vi "Get Motor Setpoint Value.vi"(8 "error in (no error)":errorcluster, 10 "state mode":T1 items=["undefined", "angle", "velocity"], 11 "motor communication in":refnum<class "NI_Robotics_Motor Communication Ref.lvclass">) -> (0 "error out":errorcluster, 1 "failed?":bool, 2 "value":dbl, 3 "motor communication out":refnum<class "NI_Robotics_Motor Communication Ref.lvclass">)   [LabVIEW 2017, in "NI_Robotics_Motor Communication Ref.lvclass"]
uses:
  <vilib>/robotics/Actuation/Motor Communication Ref/NI_Robotics_Motor Communication Ref.lvclass
  <vilib>/robotics/Actuation/Motor Communication/Motor State Mode.ctl
  <vilib>/robotics/Actuation/Motor Communication Ref/NI_Robotics_Motor Communication Ref.lvclass/NI_Robotics_Motor Communication Ref.ctl
  <vilib>/robotics/Actuation/Motor Communication/Read from Motor State.vi
  <vilib>/robotics/Actuation/Motor Communication/NI_Robotics_Motor Communication.lvclass
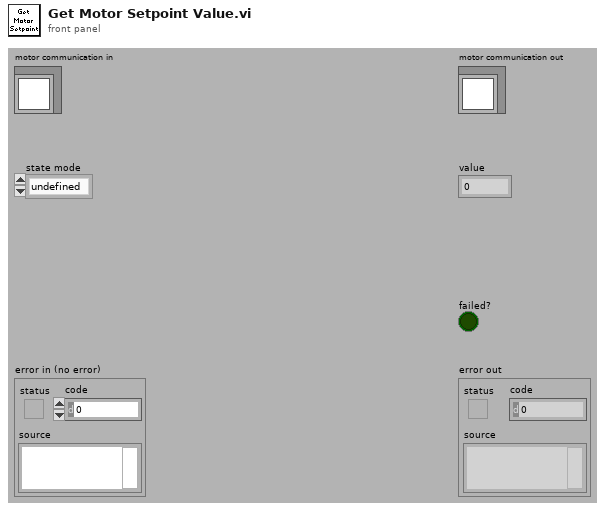
[diagram p1: front panel]
types:
  T1 = typedef "NI_Robotics_Motor Communication.lvclass/Motor State Mode.ctl" = u16
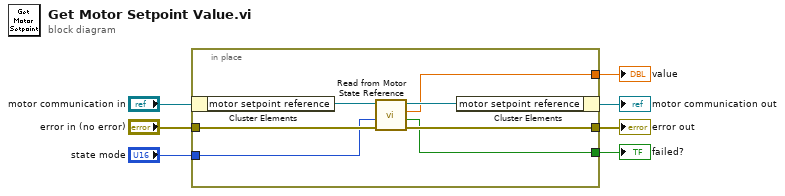
[diagram p0: block diagram]
diagram:
  n1 = in-place {
    in-place-border: [w12] -> w5
    in-place-border: "error in (no error)" -> [w11]
    in-place-border: [w10] -> w3
    in-place-border: [w9] -> w2
    in-place-border: "state mode" -> [w8]
    n2 = in-place-cluster #1("motor communication in") -> ("motor setpoint reference"=w14:refnum<data-value>)
    n3 = call <vilib>:"Read from Motor State Reference.vi"("error in (no error)"=w11, "state mode"=w8, "motor state ref in"=w14) -> ("error out"=w10:errorcluster, "failed?"=w9:bool, "value"=w12:dbl, "motor state ref out"=w13:refnum<data-value>)  [unwired: 5 in]
    n4 = in-place-cluster #1("motor setpoint reference"=w13) -> (→"motor communication out":refnum<class "NI_Robotics_Motor Communication Ref.lvclass">)
  }
  "error out" <- w3
  "failed?" <- w2
  "value" <- w5
